vi "DSF.Common.Constants.Library Name.vi"() -> (3 "Library Name":string)   [LabVIEW 2016, in "DSF.Common.lvlib"]
uses:
  DSF.Common.lvlib
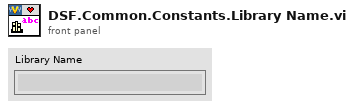
[diagram p1: front panel]
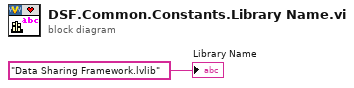
[diagram p0: block diagram]
diagram:
  "Library Name" <- "Data Sharing Framework.lvlib" ("Library Name")
